vi "Z900_navX_Internal_Close.vi"(8 "error in (no error)":errorcluster, 10 "Interface TypeDefs":T3 {"I2CDevRef"."Device Address" format="%.0x"}, 11 "navX Device":T1={"Interface"={"Protocol"=enum."SERIAL", "Update Rate (4Hz-100Hz)"=4, "navX Open TypeDef"=variant}, "Notify Packet"=refnum, "Loop VI Refnum"=refnum, "Ready to Close Occurrence Refnum"=refnum} {"Interface"."Update Rate (4Hz-100Hz)" min=4 max=60 step=1}) -> (0 "error out":errorcluster, 3 "navX Device":T1={"Interface"={"Protocol"=enum."SERIAL", "Update Rate (4Hz-100Hz)"=4, "navX Open TypeDef"=variant}, "Notify Packet"=refnum, "Loop VI Refnum"=refnum, "Ready to Close Occurrence Refnum"=refnum} {"Interface"."Update Rate (4Hz-100Hz)" min=4 max=60 step=1})   [LabVIEW 2017, in "navX Library v2.lvlib"]
doc: "This navX VI handles closing the Serial/I2C/SPI reference for the navX.\nTHIS VI SHOULD NOT BE CALLED BY THE USER!"
uses:
  navX Library v2.lvlib
  TypeDefs/Z900_navX_DeviceTypeDef.ctl
  TypeDefs/Z900_navX_ProtocolTypeDef.ctl
  TypeDefs/Z900_navX_NotifyPacketTypeDef.ctl
  TypeDefs/Z900_navX_ActionTypeDef.ctl
  TypeDefs/Z900_navX_InterfaceTypeDef.ctl
  <vilib>/Rock Robotics/WPI/SerialPort/WPI_SerialPortRef.ctl
  <vilib>/Rock Robotics/WPI/I2C/WPI_I2CDevRef.ctl
  <vilib>/Rock Robotics/SystemInterfaces/i2clib/i2c_bus.ctl
  <vilib>/Rock Robotics/WPI/SPI/WPI_SPIDevRef.ctl
  <vilib>/Rock Robotics/SystemInterfaces/spilib/spi_bus.ctl
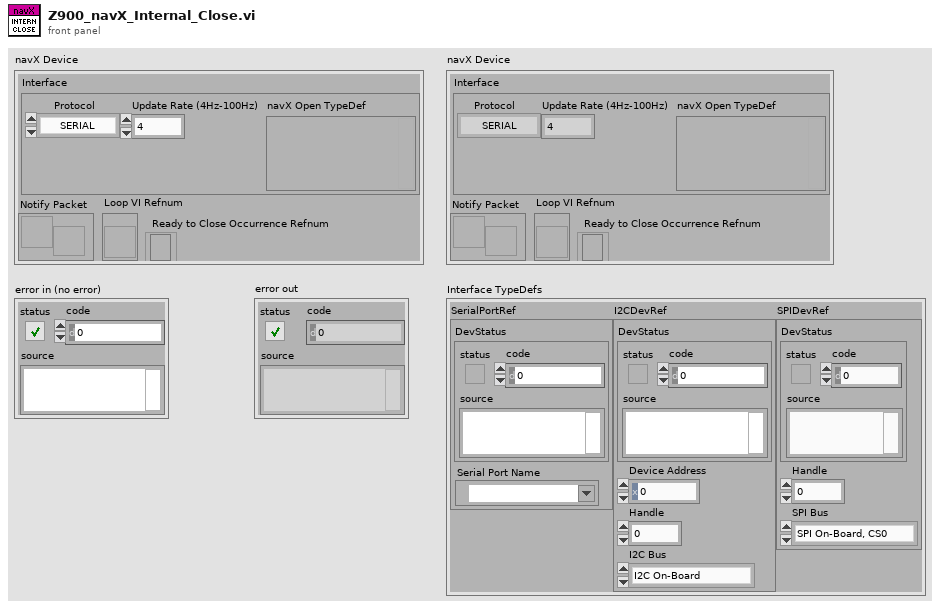
[diagram p1: front panel]
types:
  T1 = typedef "navX Library v2.lvlib/Z900_navX_DeviceTypeDef.ctl" = cluster{"Interface":cluster{"Protocol":T2, "Update Rate (4Hz-100Hz)":u8, "navX Open TypeDef":variant}, "Notify Packet":refnum<notifier>, "Loop VI Refnum":refnum<vi>, "Ready to Close Occurrence Refnum":refnum<k4>}
  T2 = typedef "navX Library v2.lvlib/Z900_navX_ProtocolTypeDef.ctl" = enum16{"SERIAL", "I2C", "SPI"}
  T3 = typedef "navX Library v2.lvlib/Z900_navX_InterfaceTypeDef.ctl" = cluster{"SerialPortRef":T4, "I2CDevRef":T5, "SPIDevRef":T7}
  T4 = typedef "WPI_SerialPortRef.ctl" = cluster{"DevStatus":errorcluster, "Serial Port Name":refnum<visa-resource-name>}
  T5 = typedef "WPI_I2CDevRef.ctl" = cluster{"DevStatus":errorcluster, "Device Address":u8, "Handle":i32, "I2C Bus":T6}
  T6 = typedef "i2c_bus.ctl" = enum16{"I2C On-Board", "I2C MXP", "Invalid"}
  T7 = typedef "WPI_SPIDevRef.ctl" = cluster{"DevStatus":errorcluster, "Handle":i32, "SPI Bus":T8}
  T8 = typedef "spi_bus.ctl" = enum16{"SPI On-Board, CS0", "SPI On-Board, CS1", "SPI On-Board, CS2", "SPI On-Board, CS3", "SPI MXP", "Invalid"}
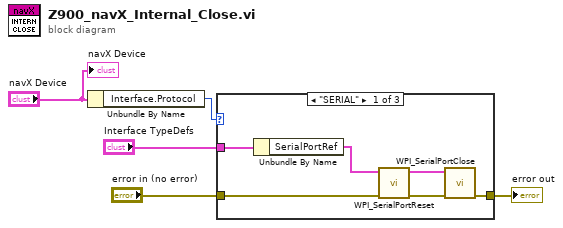
[diagram p0: block diagram]
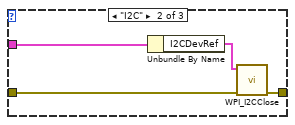
[diagram p2: hidden frame]
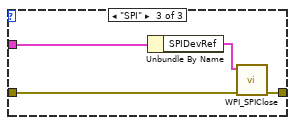
[diagram p3: hidden frame]
diagram:
  n1 = Unbundle By Name("navX Device") -> ("Interface.Protocol"=w3:T2)
  n2 = case shown="\"SERIAL\"" w3 {
    tunnel: "Interface TypeDefs" -> [w11 w15 w19]
    tunnel: [w10 w13 w17] -> w5
    tunnel: "error in (no error)" -> [w8 w12 w16]
    frame "SERIAL" {
      n3 = Unbundle By Name(w11) -> ("SerialPortRef"=w9:T4)
      n4 = call <vilib>:"WPI_SerialPortReset.vi"("error in (no error)"=w8, "SerialPortRef"=w9) -> ("error out"=w6:errorcluster, "SerialPortRef"=w7:T4)  [unwired: 8 in]
      n5 = call <vilib>:"WPI_SerialPortClose.vi"("error in (no error)"=w6, "SerialPortRef"=w7) -> ("error out"=w10:errorcluster)  [unwired: 9 in]
    }
    frame "I2C" {
      n6 = Unbundle By Name(w15) -> ("I2CDevRef"=w14:T5)
      n7 = call <vilib>:"WPI_I2CClose.vi"("error in (no error)"=w12, "I2CDevRef"=w14) -> ("error out"=w13:errorcluster)  [unwired: 9 in]
    }
    frame "SPI" {
      n8 = Unbundle By Name(w19) -> ("SPIDevRef"=w18:T7)
      n9 = call <vilib>:"WPI_SPIClose.vi"("error in (no error)"=w16, "SPIDevRef"=w18) -> ("error out"=w17:errorcluster)  [unwired: 9 in]
    }
  }
  "error out" <- w5
  "navX Device" <- "navX Device"
